vi "Electrode Switch Function.vi"(0 "LINX Resource":T1, 1 "On-time (ms)":u32, 2 "Frequency":u32, 3 "Pin Number":u8, 4 "On or Off?":bool, 5 "Error In":errorcluster, 6 "User Prompts Ref":refnum<vi>, 7 "DC or AC?":bool, 8 "Electrode Control":refnum<vi>, 9 "Row":i32, 11 "Column":i32) -> (14 "LINX Resource Out":T1, 19 "Error Out":errorcluster)   [LabVIEW 2017]
uses:
  <vilib>/MakerHub/LINX/Private/Type Defs/LINX Ref.ctl
  <vilib>/MakerHub/LINX/Private/Type Defs/Platform.ctl
  <vilib>/MakerHub/LINX/Private/Type Defs/Interface.ctl
  <vilib>/MakerHub/LINX/Private/Device/Type Defs/LINX Device Config.ctl
  <vilib>/MakerHub/LINX/Private/Device/Type Defs/TCP Config.ctl
  <vilib>/MakerHub/LINX/Private/Device/Type Defs/Channels.ctl
  <vilib>/MakerHub/LINX/Public/Peripherals/Digital/Digital Write 1 Chan.vi
  <vilib>/MakerHub/LINX/Public/Peripherals/Digital/Digital Write N Chans.vi
  <vilib>/MakerHub/LINX/Private/Local IO/LinxDigitalWrite.vi
  <vilib>/MakerHub/LINX/Public/Utilities/Check Channel.vi
  <vilib>/MakerHub/LINX/Private/Utilties/Generate Error.vi
  <vilib>/MakerHub/LINX/LMH-LINX.lvlib
  <vilib>/MakerHub/LINX/Private/Device/Device.lvlib
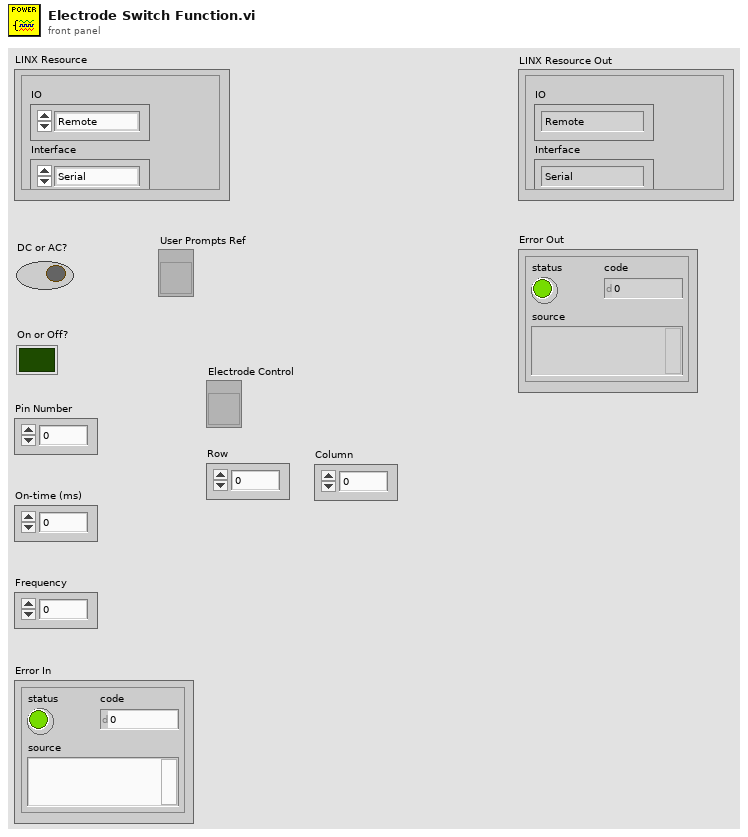
[diagram p1: front panel]
types:
  T1 = typedef "LMH-LINX.lvlib/LINX Ref.ctl" = cluster{"IO":T2, "Interface":T3, "LINX Device Config":T4}
  T2 = typedef "LMH-LINX.lvlib/Platform.ctl" = enum16{"Remote", "Local"}
  T3 = typedef "LMH-LINX.lvlib/Interface.ctl" = enum16{"Serial", "TCP"}
  T4 = typedef "LMH-LINX.lvlib/Device.lvlib/LINX Device Config.ctl" = cluster{"Interface":T3, "COM Port":refnum<visa-resource-name>, "TCP Configuration":T5, "Device Family":u8, "Device ID":u8, "Device Name":string, "TCP Ref":refnum<k5>, "Channels":T6}
  T5 = typedef "LMH-LINX.lvlib/Device.lvlib/TCP Config.ctl" = cluster{"IP Address":string, "Port":u16}
  T6 = typedef "LMH-LINX.lvlib/Channels.ctl" = cluster{"DI":u8[], "DO":u8[], "AI":u8[], "AO":u8[], "PWM":u8[], "QE":u8[], "UART":u8[], "I2C 2":u8[], "SPI":u8[], "CAN":u8[], "Servo":u8[], "AI Ref (V)":dbl, "AI Resolution (Bits)":u8, "AO Ref (V)":dbl, "AO Resolution (Bits)":u8}
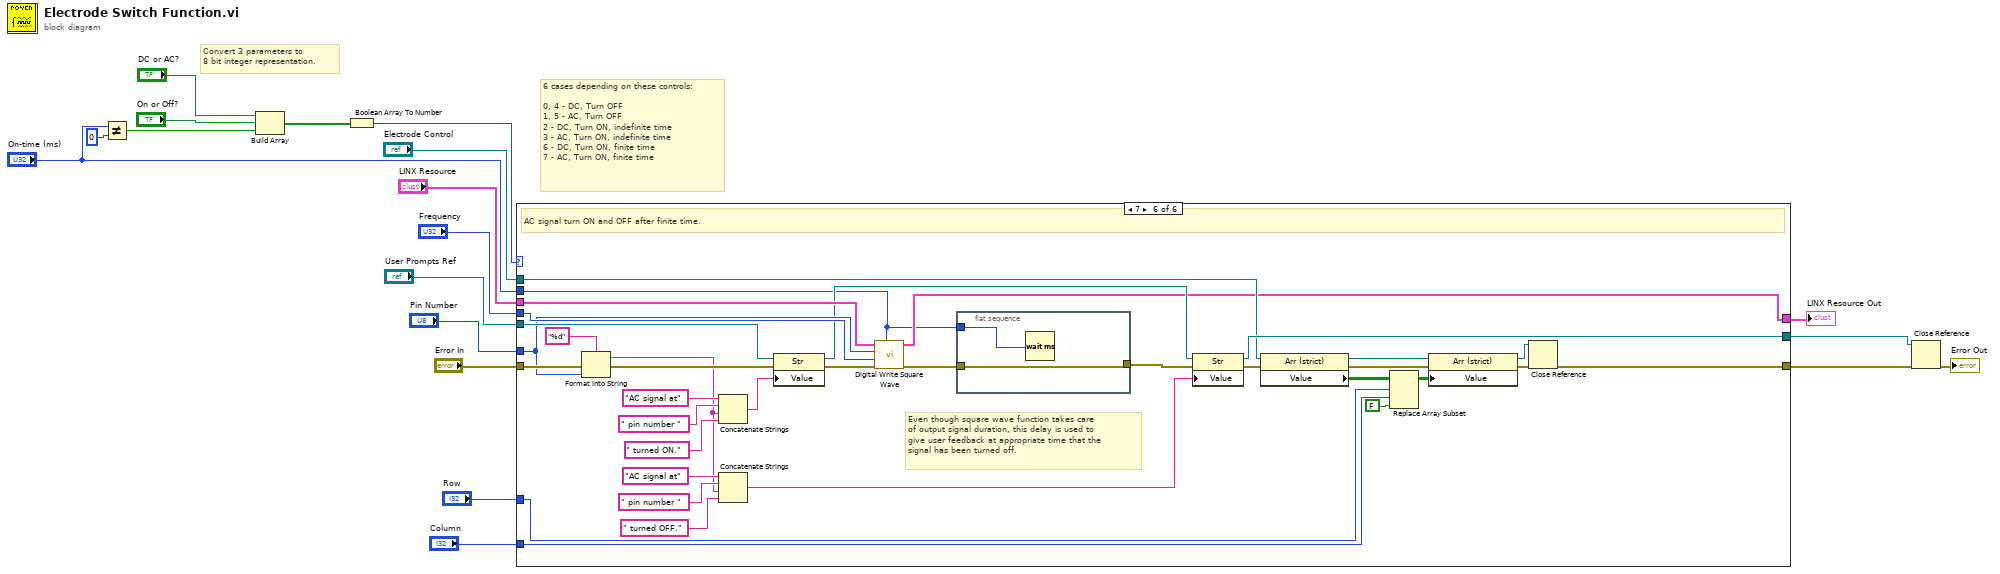
[diagram p0: block diagram]
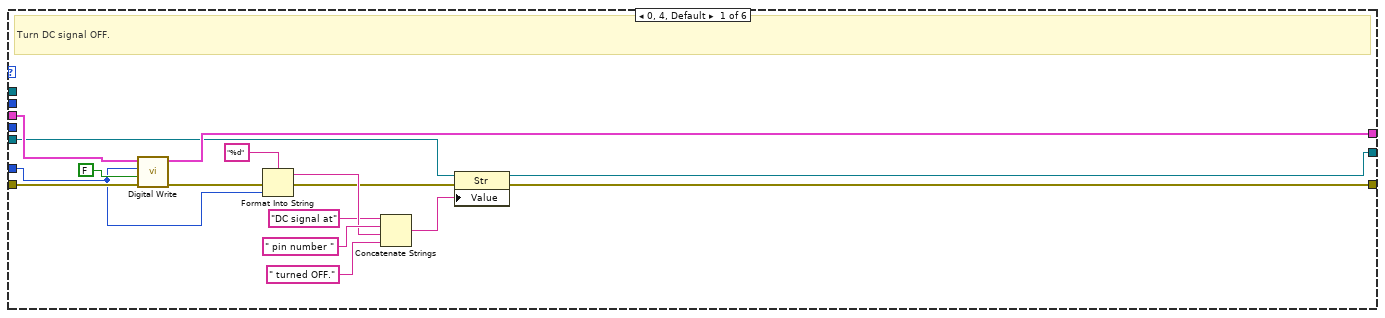
[diagram p2: hidden frame]
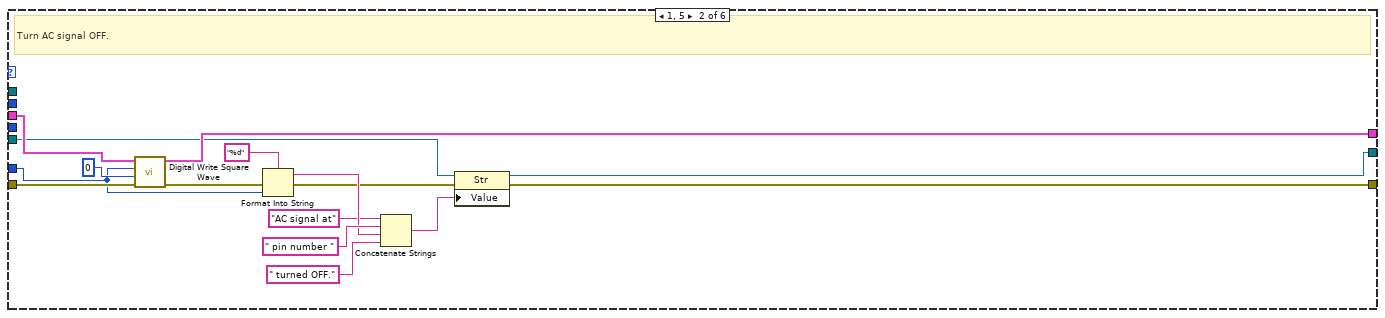
[diagram p3: hidden frame]
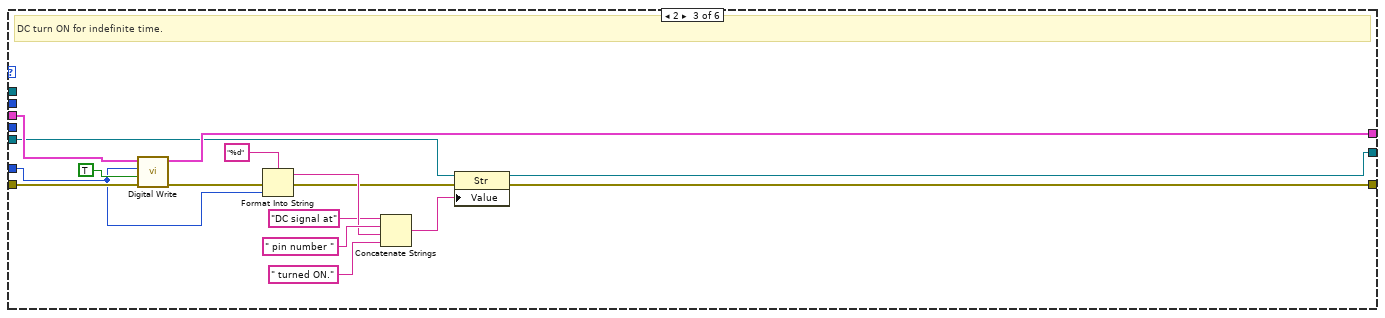
[diagram p4: hidden frame]
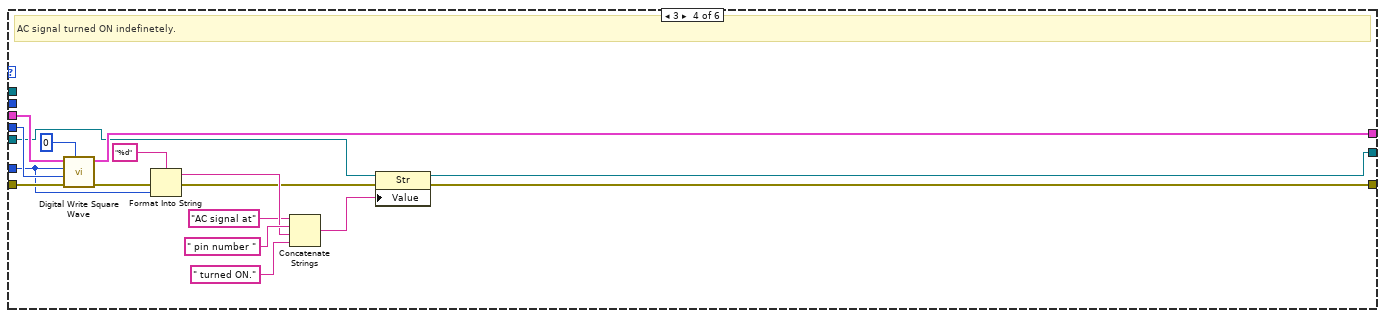
[diagram p5: hidden frame]
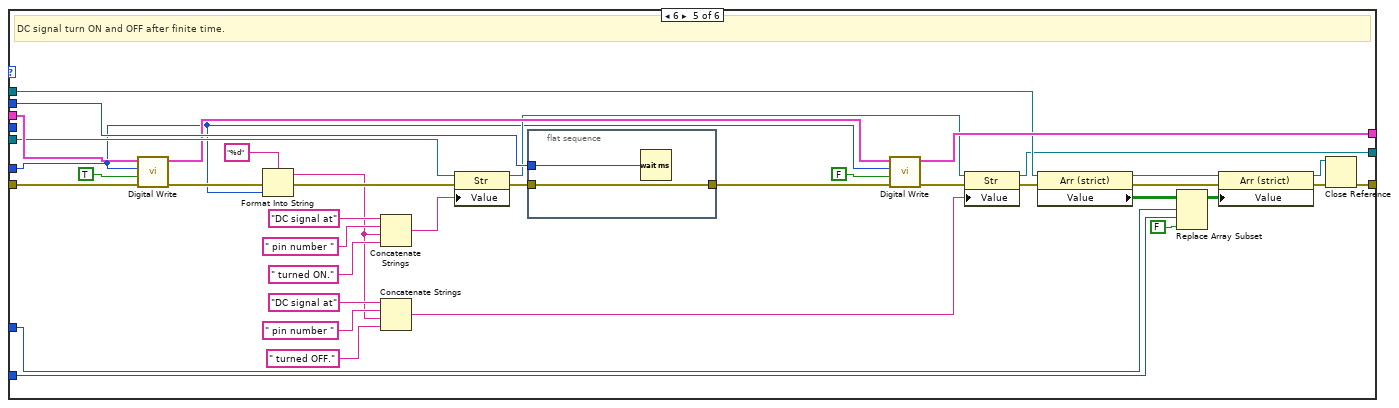
[diagram p6: hidden frame]
diagram:
  # "Convert 3 parameters to\n8 bit integer representation."
  # "6 cases depending on these controls:\n\n0, 4 - DC, Turn OFF\n1, 5 - AC, Turn OFF\n2 - DC, Turn ON, indefinite time\n3 - AC, Turn ON, indefinite time\n6 - DC, Turn ON, finite time\n7 - AC, Turn ON, finite time"
  n1 = Not Equal?(x="On-time (ms)", y=u32 0) -> (x != y?=w16:bool)
  n2 = Build Array("DC or AC?", "On or Off?", w16) -> (w15:bool[])
  n3 = Boolean Array To Number(Boolean array=w15) -> (number=w14:u32)
  n4 = case shown="7" w14 {
    tunnel: "Error In" -> [w33 w51 w66 w84 w122 w152]
    tunnel: "LINX Resource" -> [w35 w50 w67 w82 w121 w148]
    tunnel: "User Prompts Ref" -> [w31 w39 w56 w71 w112 w153]
    tunnel: "Pin Number" -> [w30 w40 w53 w68 w101 w149]
    tunnel: "Frequency" -> [_ _ _ w83 _ w150]
    tunnel: [w34 w49 w57 w80 w106 w128] -> w8
    tunnel: [w21 w38 w54 w69 w88 w134] -> w7
    tunnel: [w22 w37 w55 w70 w85 w129] -> w6
    tunnel: "On-time (ms)" -> [_ _ _ _ w111 w127]
    tunnel: "Electrode Control" -> [_ _ _ _ w96 w132]
    tunnel: "Row" -> [_ _ _ _ w94 w131]
    tunnel: "Column" -> [_ _ _ _ w93 w130]
    frame 0, 4, Default {
      # "Turn DC signal OFF."
      n5 = call-poly <vilib>:"Digital Write.vi"("Error In"=w33, "Output Value"=FALSE, "DO Channel"=w30, "LINX Resource"=w35) -> ("Error Out"=w28:errorcluster, "LINX Resource"=w34:T1)  [unwired: 6 in]
      n6 = Format Into String(format string="%d", error in=w28, w30) -> (resulting string=w26:string, error out=w23:errorcluster)  [unwired: 1 in]
      n7 = Concatenate Strings("DC signal at" ("string"), " pin number " ("string"), w26, " turned OFF." ("string")) -> (w24:string)
      n8 = property class="Str"(reference=w31, error in=w23, "Value"=w24) -> (reference out=w21:refnum<vi>, error out=w22:errorcluster)
    }
    frame 1, 5 {
      # "Turn AC signal OFF."
      n9 = call <vilib>:"Digital Write Square Wave.vi"("Error In"=w51, "Frequency (Hz)"=u32 0, "Channel"=w40, "LINX Resource"=w50) -> ("Error Out"=w41:errorcluster, "LINX Resource"=w49:T1)  [unwired: 6 in]
      n10 = Format Into String(format string="%d", error in=w41, w40) -> (resulting string=w45:string, error out=w42:errorcluster)  [unwired: 1 in]
      n11 = Concatenate Strings("AC signal at" ("string"), " pin number " ("string"), w45, " turned OFF." ("string")) -> (w43:string)
      n12 = property class="Str"(reference=w39, error in=w42, "Value"=w43) -> (reference out=w38:refnum<vi>, error out=w37:errorcluster)
    }
    frame 2 {
      # "DC turn ON for indefinite time."
      n13 = call-poly <vilib>:"Digital Write.vi"("Error In"=w66, "Output Value"=TRUE, "DO Channel"=w53, "LINX Resource"=w67) -> ("Error Out"=w58:errorcluster, "LINX Resource"=w57:T1)  [unwired: 6 in]
      n14 = Format Into String(format string="%d", error in=w58, w53) -> (resulting string=w62:string, error out=w59:errorcluster)  [unwired: 1 in]
      n15 = Concatenate Strings("DC signal at" ("string"), " pin number " ("string"), w62, " turned ON." ("string")) -> (w60:string)
      n16 = property class="Str"(reference=w56, error in=w59, "Value"=w60) -> (reference out=w54:refnum<vi>, error out=w55:errorcluster)
    }
    frame 3 {
      # "AC signal turned ON indefinetely."
      n17 = call <vilib>:"Digital Write Square Wave.vi"("Duration (ms)"=u32 0, "Error In"=w84, "Frequency (Hz)"=w83, "Channel"=w68, "LINX Resource"=w82) -> ("Error Out"=w72:errorcluster, "LINX Resource"=w80:T1)  [unwired: 5 in]
      n18 = Format Into String(format string="%d", error in=w72, w68) -> (resulting string=w77:string, error out=w74:errorcluster)  [unwired: 1 in]
      n19 = Concatenate Strings("AC signal at" ("string"), " pin number " ("string"), w77, " turned ON." ("string")) -> (w75:string)
      n20 = property class="Str"(reference=w71, error in=w74, "Value"=w75) -> (reference out=w69:refnum<vi>, error out=w70:errorcluster)
    }
    frame 6 {
      # "DC signal turn ON and OFF after finite time."
      n21 = call-poly <vilib>:"Digital Write.vi"("Error In"=w122, "Output Value"=TRUE, "DO Channel"=w101, "LINX Resource"=w121) -> ("Error Out"=w113:errorcluster, "LINX Resource"=w108:T1)  [unwired: 6 in]
      n22 = Format Into String(format string="%d", error in=w113, w101) -> (resulting string=w99:string, error out=w115:errorcluster)  [unwired: 1 in]
      n23 = Concatenate Strings("DC signal at" ("string"), " pin number " ("string"), w99, " turned ON." ("string")) -> (w116:string)
      n24 = Concatenate Strings("DC signal at" ("string"), " pin number " ("string"), w99, " turned OFF." ("string")) -> (w104:string)
      n25 = property class="Str"(reference=w112, error in=w115, "Value"=w116) -> (reference out=w102:refnum<vi>, error out=w110:errorcluster)
      n26 = flat-sequence {
        tunnel: w111 -> [w124]
        tunnel: w110 -> [w123]
        tunnel: [w123] -> w109
        frame #0 {
          n27 = Wait (ms)(milliseconds to wait=w124) -> ()  [unwired: 1 out]
        }
      }
      n28 = call-poly <vilib>:"Digital Write.vi"("Error In"=w109, "Output Value"=FALSE, "DO Channel"=w101, "LINX Resource"=w108) -> ("Error Out"=w100:errorcluster, "LINX Resource"=w106:T1)  [unwired: 6 in]
      n29 = property class="Str"(reference=w102, error in=w100, "Value"=w104) -> (reference out=w88:refnum<vi>, error out=w97:errorcluster)
      n30 = property class="Arr (strict)"(reference=w96, error in=w97) -> (reference out=w91:refnum<vi>, error out=w90:errorcluster, "Value"=w95:bool[][])
      n31 = Replace Array Subset(array=w95, new element=FALSE ("new element/subarray"), index (row)=w94, index (col)=w93) -> (w89:bool[][])
      n32 = property class="Arr (strict)"(reference=w91, error in=w90, "Value"=w89) -> (reference out=w86:refnum<vi>, error out=w87:errorcluster)
      n33 = Close Reference(reference=w86, error in (no error)=w87) -> (error out=w85:errorcluster)
    }
    frame 7 {
      # "Even though square wave function takes care\nof output signal duration, this delay is used to\ngive user feedback at appropriate time that the \nsignal has been turned off."
      # "AC signal turn ON and OFF after finite time."
      n34 = Format Into String(format string="%d", error in=w152, w149) -> (resulting string=w142:string, error out=w155:errorcluster)  [unwired: 1 in]
      n35 = Concatenate Strings("AC signal at" ("string"), " pin number " ("string"), w142, " turned ON." ("string")) -> (w156:string)
      n36 = Concatenate Strings("AC signal at" ("string"), " pin number " ("string"), w142, " turned OFF." ("string")) -> (w145:string)
      n37 = property class="Str"(reference=w153, error in=w155, "Value"=w156) -> (reference out=w143:refnum<vi>, error out=w151:errorcluster)
      n38 = call <vilib>:"Digital Write Square Wave.vi"("Duration (ms)"=w127, "Error In"=w151, "Frequency (Hz)"=w150, "Channel"=w149, "LINX Resource"=w148) -> ("Error Out"=w126:errorcluster, "LINX Resource"=w128:T1)  [unwired: 5 in]
      n39 = flat-sequence {
        tunnel: w127 -> [w161]
        tunnel: [w160] -> w125
        tunnel: w126 -> [w160]
        frame #0 {
          n40 = Wait (ms)(milliseconds to wait=w161) -> ()  [unwired: 1 out]
        }
      }
      n41 = property class="Str"(reference=w143, error in=w125, "Value"=w145) -> (reference out=w134:refnum<vi>, error out=w133:errorcluster)
      n42 = property class="Arr (strict)"(reference=w132, error in=w133) -> (reference out=w139:refnum<vi>, error out=w138:errorcluster, "Value"=w141:bool[][])
      n43 = Replace Array Subset(array=w141, new element=FALSE ("new element/subarray"), index (row)=w131, index (col)=w130) -> (w137:bool[][])
      n44 = property class="Arr (strict)"(reference=w139, error in=w138, "Value"=w137) -> (reference out=w135:refnum<vi>, error out=w136:errorcluster)
      n45 = Close Reference(reference=w135, error in (no error)=w136) -> (error out=w129:errorcluster)
    }
  }
  "LINX Resource Out" <- w8
  n46 = Close Reference(reference=w7, error in (no error)=w6) -> (error out=→"Error Out":errorcluster)
